vi "VI-Create Refs From Controls.vi"(0 "TopLevelDiagram in":refnum<vi>, 7 "SelList[]":refnum<vi>[](array[refnum]), 11 "error in (no error)":errorcluster) -> (6 "Ref refs":refnum<vi>[](array[refnum]), 8 "X":u32, 10 "Y":i32, 14 "Names":string[](array[string]), 15 "error out":errorcluster)   [LabVIEW 2015]
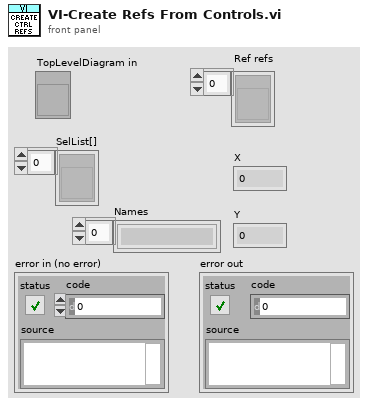
[diagram p1: front panel]
types:
  T1 = cluster{"Object Label":string, "dup GObject":refnum<vi>}
  T2 = cluster{"Object Label":string, "dup GObject":refnum<vi>}[]
  T3 = typedef "LVRectTypeDef.ctl" = cluster{"Left":i16, "Top":i16, "Right":i16, "Bottom":i16}
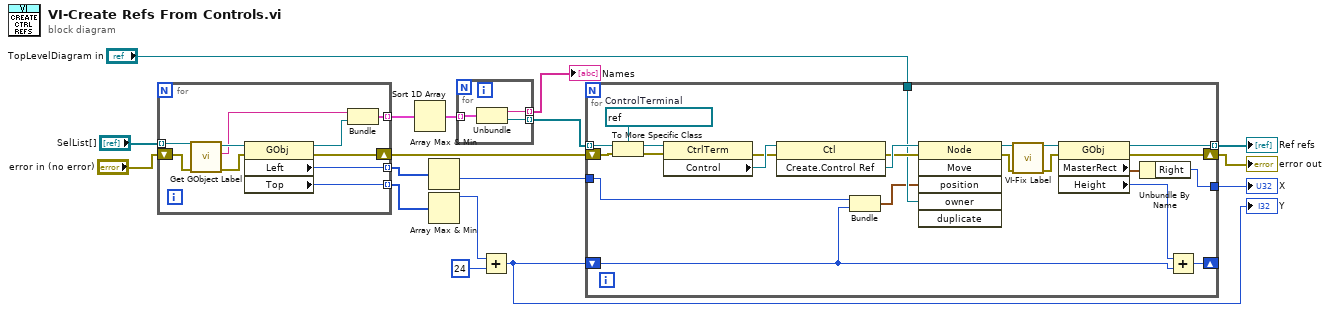
[diagram p0: block diagram]
diagram:
  n1 = for {
    tunnel: "SelList[]" -> [w27] mode=indexing
    shift-right: [w25] -> w15
    shift-left: "error in (no error)" -> [w26]
    tunnel: [w22] -> w7 mode=indexing
    tunnel: [w21] -> w13 mode=indexing
    tunnel: [w18] -> w5 mode=indexing
    n2 = call <vilib>:"Get GObject Label.vi"("error in (no error)"=w26, "GObject"=w27) -> ("error out"=w24:errorcluster, "Object Label"=w20:string, "dup GObject"=w23:refnum<vi>)  [unwired: 5 in, 2 out]
    n3 = property class="GObj"(reference=w23, error in=w24) -> (reference out=w19:refnum<vi>, error out=w25:errorcluster, "Left"=w22:i32, "Top"=w21:i32)
    n4 = Bundle("Object Label"=w20, "dup GObject"=w19) -> (w18:T1)  [unwired: 1 in]
  }
  n5 = Sort 1D Array(array=w5) -> (sorted array=w6:T2)
  n6 = Array Max & Min(array=w7) -> (min value=w12:i32)  [unwired: 3 out]
  n7 = Array Max & Min(array=w13) -> (max value=w11:i32)  [unwired: 3 out]
  n8 = for {
    tunnel: w6 -> [w30] mode=indexing
    tunnel: [w29] -> w8 mode=indexing
    tunnel: [w28] -> w3 mode=indexing
    n9 = Unbundle(w30) -> ("Object Label"=w28:string, "dup GObject"=w29:refnum<vi>)
  }
  "Names" <- w3
  n10 = Add(x=w11, y=24) -> (x+y=w14:i32)
  "Y" <- w14
  n11 = for {
    tunnel: "TopLevelDiagram in" -> [w48]
    tunnel: w8 -> [w52] mode=indexing
    shift-right: [w42] -> w16
    shift-left: w15 -> [w53]
    tunnel: w12 -> [w32]
    shift-right: [w41] -> _
    shift-left: w14 -> [w40]
    tunnel: [w35] -> w17 mode=indexing
    tunnel: [w31] -> w4
    w51 = refnum<vi> refnum  # ControlTerminal
    n12 = To More Specific Class(target class=w51, reference=w52, error in=w53) -> (specific class reference=w47:refnum<vi>, error out=w45:errorcluster)
    n13 = property class="CtrlTerm"(reference=w47, error in=w45) -> (error out=w44:errorcluster, "Control"=w46:refnum<vi>)  [unwired: 1 out]
    n14 = invoke class="Ctl" method="Create.Control Ref"(reference=w46, error in=w44) -> (error out=w49:errorcluster, "Create Control Ref"=w50:refnum<vi>)  [unwired: 1 in, 1 out]
    n15 = Bundle(w32, w40) -> (w43:cluster{i32, u32})  [unwired: 1 in]
    n16 = invoke class="Node" method="Move"(reference=w50, error in=w49, "position"=w43, "owner"=w48) -> (reference out=w39:refnum<vi>, error out=w37:errorcluster)  [unwired: 2 in, 4 out]
    n17 = call "VI-Fix Label.vi"("GObject in"=w39, "error in (no error)"=w37) -> ("GObject out"=w38:refnum<vi>, "error out"=w36:errorcluster)  [unwired: 12 in]
    n18 = property class="GObj"(reference=w38, error in=w36) -> (reference out=w35:refnum<vi>, error out=w42:errorcluster, "MasterRect"=w33:T3, "Height"=w34:u32)
    n19 = Unbundle By Name(w33) -> ("Right"=w31:i16)
    n20 = Add(x=w34, y=w40) -> (x+y=w41:u32)
  }
  "X" <- w4
  "Ref refs" <- w17
  "error out" <- w16
